vi "initialVI.vi"(11 "Input cluster":T1) -> (0 "Max No. of Tests":i32, 1 "Voltage/(g/s)":bool, 2 "Queue cluster":T1, 3 "Test Param":T2)   [LabVIEW 2014]
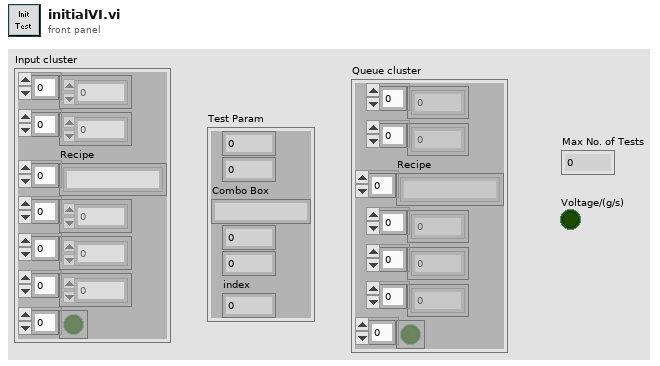
[diagram p1: front panel]
types:
  T1 = cluster{i32[], i32[], "Recipe":string[], i32[], i32[], i32[], bool[]}
  T2 = cluster{i32, i32, "Combo Box":string, i32, i32, "index":i32}
  T3 = cluster{i32, i32, "String":string, i32, i32, "index":i32}
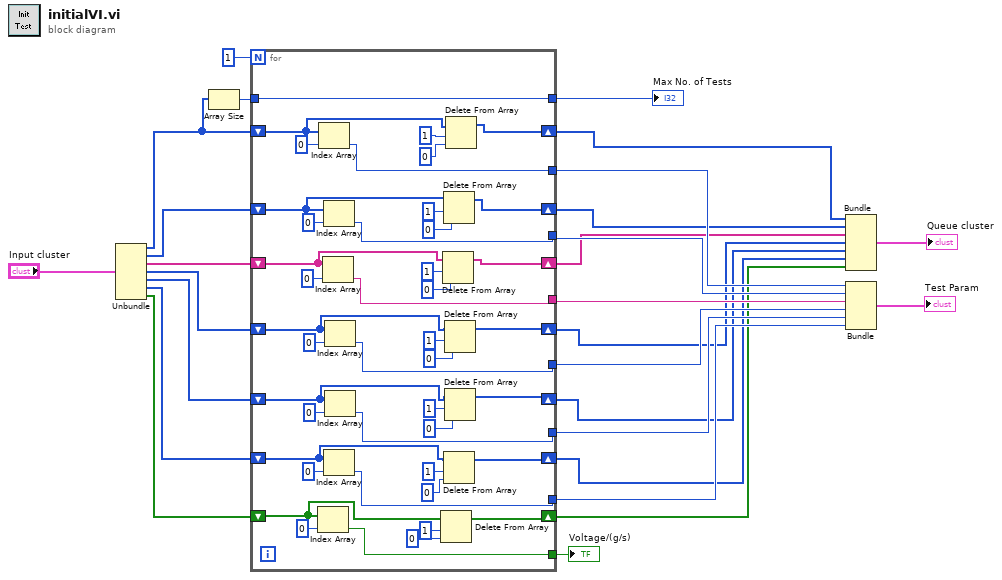
[diagram p0: block diagram]
diagram:
  n1 = Unbundle("Input cluster") -> (w8:i32[], w26:i32[], "Recipe"=w25:string[], w24:i32[], w23:i32[], w22:i32[], w4:bool[])
  n2 = Array Size(array=w8) -> (size(s)=w7:i32)
  n3 = for {
    N: 1 -> [_]
    shift-right: [w66] -> w14
    shift-left: w8 -> [w67]
    shift-right: [w35] -> w13
    shift-left: w26 -> [w55]
    shift-right: [w36] -> w12
    shift-left: w25 -> [w51]
    shift-right: [w39] -> w11
    shift-left: w24 -> [w48]
    shift-right: [w38] -> w10
    shift-left: w23 -> [w45]
    shift-right: [w37] -> w9
    shift-left: w22 -> [w42]
    tunnel: [w52] -> w20
    tunnel: [w60] -> w21
    tunnel: [w59] -> w19
    tunnel: [w58] -> w18
    tunnel: [w57] -> w17
    tunnel: [w56] -> w16
    tunnel: w7 -> [w34]
    tunnel: [w34] -> w6
    shift-right: [w29] -> w3
    shift-left: w4 -> [w32]
    tunnel: [w28] -> w1
    n4 = Index Array(array=w32, index=0) -> (element=w28:bool)
    n5 = Index Array(array=w67, index=0) -> (element=w60:i32)
    n6 = Index Array(array=w51, index=0) -> (element=w59:string)
    n7 = Index Array(array=w55, index=0) -> (element=w52:i32)
    n8 = Index Array(array=w42, index=0) -> (element=w56:i32)
    n9 = Index Array(array=w48, index=0) -> (element=w58:i32)
    n10 = Index Array(array=w45, index=0) -> (element=w57:i32)
    n11 = Delete From Array(array=w32, length=1, index=0) -> (array with subset deleted=w29:bool[])  [unwired: 1 out]
    n12 = Delete From Array(array=w51, length=1, index=0) -> (array with subset deleted=w36:string[])  [unwired: 1 out]
    n13 = Delete From Array(array=w55, length=1, index=0) -> (array with subset deleted=w35:i32[])  [unwired: 1 out]
    n14 = Delete From Array(array=w42, length=1, index=0) -> (array with subset deleted=w37:i32[])  [unwired: 1 out]
    n15 = Delete From Array(array=w48, length=1, index=0) -> (array with subset deleted=w39:i32[])  [unwired: 1 out]
    n16 = Delete From Array(array=w45, length=1, index=0) -> (array with subset deleted=w38:i32[])  [unwired: 1 out]
    n17 = Delete From Array(array=w67, length=1, index=0) -> (array with subset deleted=w66:i32[])  [unwired: 1 out]
  }
  "Max No. of Tests" <- w6
  "Voltage/(g/s)" <- w1
  n18 = Bundle(w14, w13, "Recipe"=w12, w11, w10, w9, w3) -> (→"Queue cluster":T1)  [unwired: 1 in]
  n19 = Bundle(w21, w20, "String"=w19, w18, w17, "index"=w16) -> (→"Test Param":T3)  [unwired: 1 in]
